vi "ElapsedTime.vi"(9 "error in":errorcluster, 10 "start (s)":dbl, 11 "compare time":timestamp) -> (1 "error out":errorcluster, 2 "elapsed (s)":dbl, 3 "current time":timestamp)   [LabVIEW 2013, in "MQTT Server.lvlib" / "MQTT_Base.lvclass"]
uses:
  MQTT_Base.lvclass
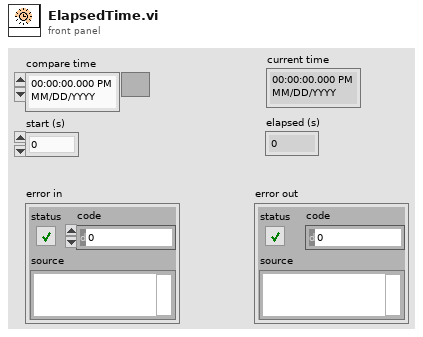
[diagram p1: front panel]
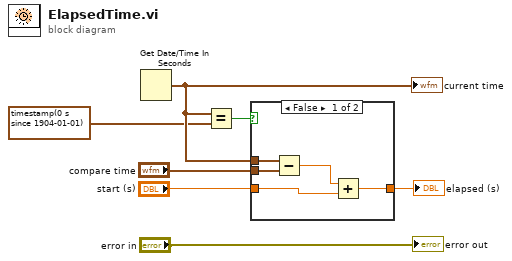
[diagram p0: block diagram]
diagram:
  n1 = Get Date/Time In Seconds() -> (seconds since 1Jan1904=w4:timestamp)
  "current time" <- w4
  n2 = Equal?(x=w4, y=timestamp(0 s since 1904-01-01)) -> (x = y?=w2:bool)
  n3 = case shown="False" w2 {
    tunnel: "compare time" -> [w12 _]
    tunnel: "start (s)" -> [w11 _]
    tunnel: [w9 _] -> w5
    tunnel: w4 -> [w8 _]
    frame False {
      n4 = Subtract(x=w8, y=w12) -> (x-y=w10:dbl)
      n5 = Add(x=w10, y=w11) -> (x+y=w9:dbl)
    }
    frame True {
    }
  }
  "elapsed (s)" <- w5
  "error out" <- "error in"
